vi "AnalogDAQ.vi"(0 "VISA resource name":refnum<visa-resource-name>="COM1", 1 "baud rate":u32=9600, 2 "data bits":u16=8 min=5 max=8 step=1, 3 "parity":u16(ring) items=["None", "Odd", "Even", "Mark", "Space"], 4 "stop bits":u16(ring)=10 items=["1.0"=10, "1.5"=15, "2.0"=20], 7 "flow control":u16(ring) items=["None"=0, "XON/XOFF"=1, "RTS/CTS"=2, "DTR/DSR"=4]) -> ()   [LabVIEW 2013]
doc: "The Basic Serial Read and Write example performs a Serial Port Read, a Serial Port Write, or a combination of these actions. The user selects the actions (read or write) on the front panel. If both are selected, the VI will write the data first, read data, and then close the VISA session that is opened to the port. This VI will wait until the specified number of bytes is received at the port. Only the number of bytes specified will be read.\n\nINSTRUCTIONS:\n1) Select the serial resource and configuration parameters (baud rate, data bits, parity, stop bits, flow control).\n2) Select the operations to be performed. \n3) Connect the serial port to your device. If no device is available, perform a loopback test by doing one of the following. Short pins 2 and 3 on a RS-232 cable or short pin 4 to pin 8 and pin 5 to pin 9 on a RS-485/422 cable. \n4) Run the VI to see the data read. (The \"read string\" will match the \"string to write\" if a loopback test was performed.)\n\nNote: The parameters set for the serial port must match the parameters of the connected instrument or device. In this example, the bytes to read parameter specifies the number of bytes that the serial port reads. If there were more bytes at the port than the number specified in bytes to read, those bytes would not be read. Also, if you specify to read more bytes than the number of bytes actually read, you might receive a timeout error message.\n\nOn the block diagram, the Configure Serial Port VI sets the configuration parameters. The front panel displays the controls used to configure the basic parameters, such as baud rate, data bits, and parity. Constants configure the other parameters the user probably does not need set. After the VISA Configure Serial Port VI opens the VISA session and configures the port, the VI passes the VISA resource name to other VIs that perform operations on that VISA resource. The VISA Write function sends a command to the serial device and the VISA Read function returns data based on the command. The VISA Close function then closes the reference to the serial device. It is important to close the reference; otherwise communication through with that port through protocols other than VISA might not be possible."
uses:
  <vilib>/Instr/_visa.llb/VISA Configure Serial Port (Instr).vi
panel:
  in  "Plot visible":bool[](array[boolean])=[TRUE, TRUE, TRUE, TRUE, TRUE, TRUE, TRUE]
  in  "stop":bool
  out "Analog Read":dbl[][](graph)
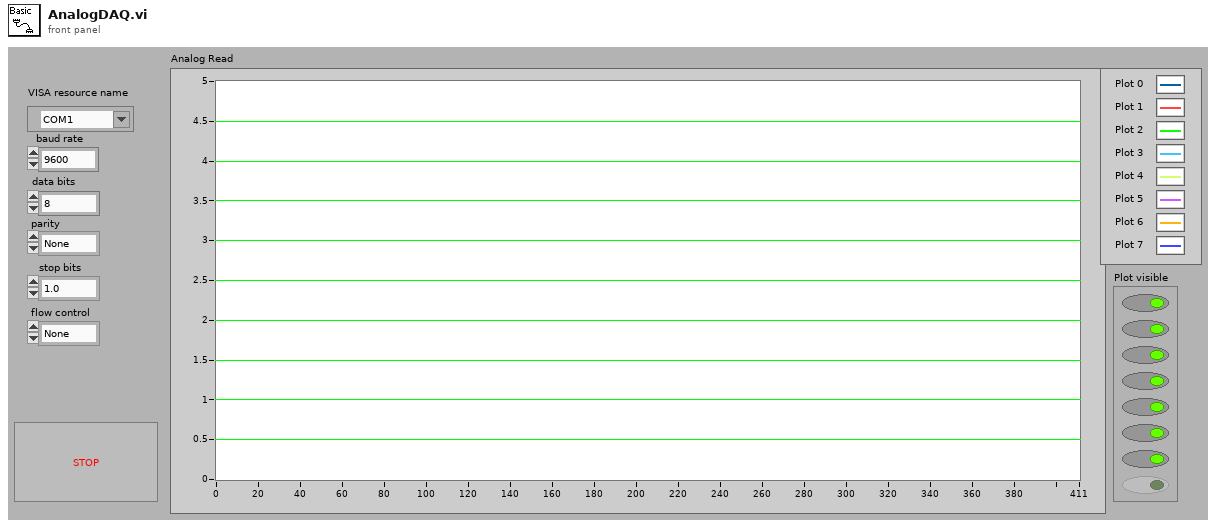
[diagram p1: front panel]
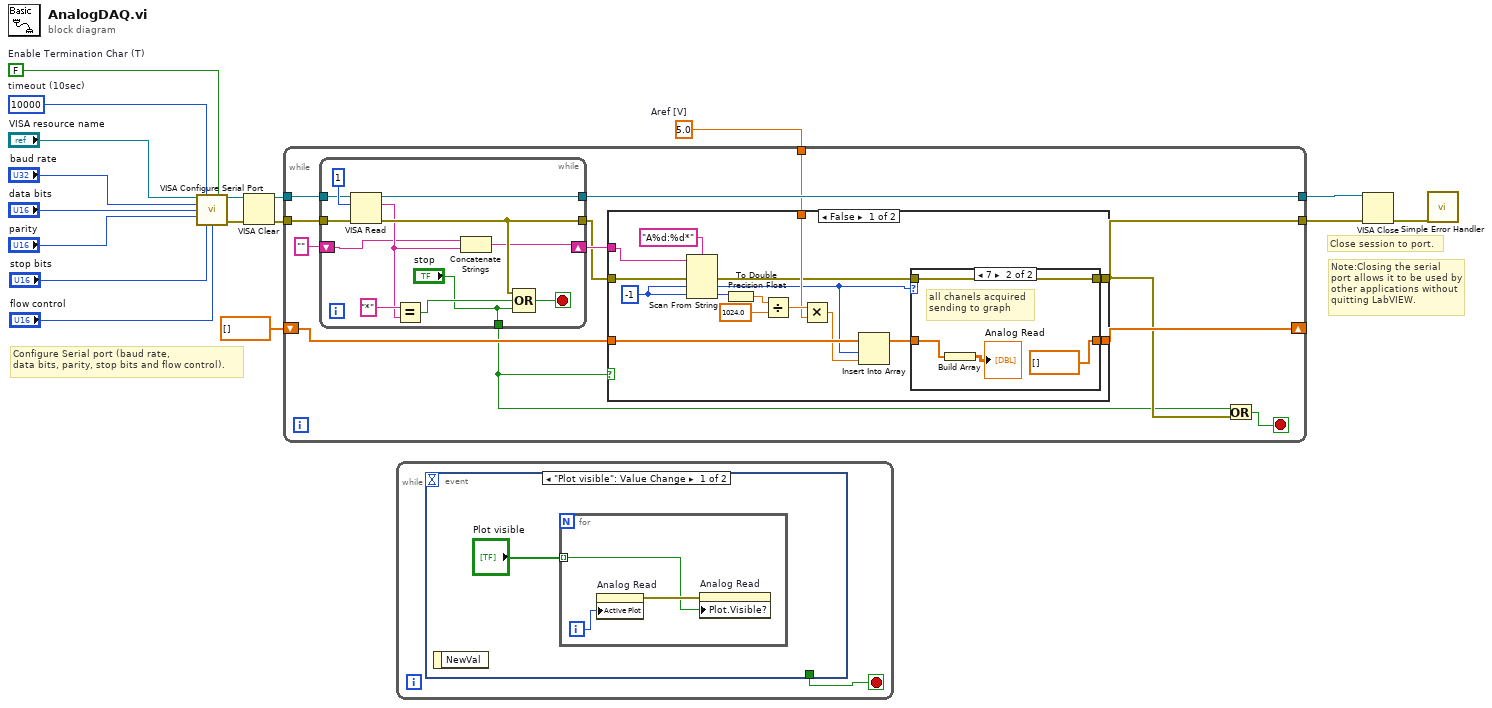
[diagram p0: block diagram]
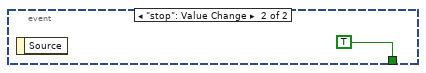
[diagram p2: hidden frame]
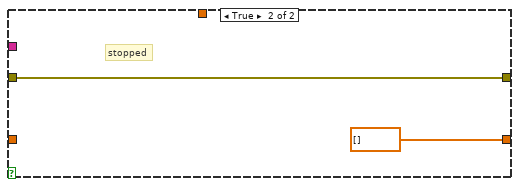
[diagram p4: hidden frame]
diagram:
  w5 = 5.0  # Aref [V]
  w12 = FALSE  # Enable Termination Char (T)
  w13 = u32 10000  # timeout (10sec)
  # "Note:Closing the serial port allows it to be used by other applications without\nquitting LabVIEW."
  # "Configure Serial port (baud rate,\ndata bits, parity, stop bits and flow control)."
  # "Close session to port."
  n1 = call-poly "VISA Configure Serial Port"("VISA resource name"="VISA resource name", "timeout (10sec)"=w13, "Enable Termination\nChar (T)"=w12, "baud rate (9600)"="baud rate", "data bits (8)"="data bits", "parity (0:none)"="parity", "stop bits (10: 1 bit)"="stop bits", "flow control (0:none)"="flow control") -> ("VISA resource name out"=w3:refnum<visa-resource-name>, "error out"=w4:errorcluster)  [unwired: 6 in]
  n2 = VISA Clear(VISA resource name=w3, error in (no error)=w4) -> (VISA resource name out=w2:refnum<visa-resource-name>, error out=w1:errorcluster)
  n3 = while {
    tunnel: [w19] -> w8
    tunnel: [w29] -> w7
    tunnel: w1 -> [w28]
    tunnel: w2 -> [w27]
    shift-right: [w20] -> _
    shift-left: dbl[] [] -> [w22]
    tunnel: w5 -> [w21]
    stop <- w25 stop-if-true
    n4 = while {
      tunnel: [w58] -> w23
      tunnel: [w65] -> w29
      tunnel: w28 -> [w63]
      tunnel: w27 -> [w62]
      shift-right: [w57] -> w24
      shift-left: "" -> [w55]
      tunnel: ["stop"] -> w18
      stop <- w59 stop-if-true
      n5 = VISA Read(VISA resource name=w62, byte count=u32 1 ("bytes to read 2"), error in (no error)=w63) -> (VISA resource name out=w65:refnum<visa-resource-name>, read buffer=w56:string, error out=w58:errorcluster)  [unwired: 1 out]
      n6 = Equal?(x="*", y=w56) -> (x = y?=w60:bool)
      n7 = Concatenate Strings(w55, w56) -> (w57:string)
      n8 = Compound Arithmetic op=OR(w58, w60, "stop") -> (w59:bool)
    }
    n9 = case shown="False" w18 {
      tunnel: w24 -> [w44 _]
      tunnel: w23 -> [w43 w52]
      tunnel: w22 -> [w41 _]
      tunnel: w21 -> [w36 _]
      tunnel: [w32 dbl[] []] -> w20
      tunnel: [w30 w52] -> w19
      frame False {
        w42 = -1 ("default value 1")
        n10 = Scan From String(format string="A%d:%d*", input string=w44, error in=w43, default 1=w42, default 2=w42) -> (error out=w31:errorcluster, output 1=w34:i32, output 2=w40:i32)  [unwired: 1 in, 2 out]
        n11 = To Double Precision Float(number=w40) -> (double precision float=w39:dbl)
        n12 = Divide(x=w39, y=1024.0) -> (x/y=w37:dbl)
        n13 = Multiply(x=w37, y=w36) -> (x*y=w35:dbl)
        n14 = Insert Into Array(array=w41, index=w34, new element=w35) -> (w33:dbl[])
        n15 = case shown="7" w34 {
          tunnel: w33 -> [w47 w48]
          tunnel: [w47 dbl[] []] -> w32
          tunnel: w31 -> [w46 w50]
          tunnel: [w46 w50] -> w30
          frame Default {
          }
          frame 7 {
            # "all chanels acquired\nsending to graph"
            n16 = Build Array(w48) -> (→"Analog Read":dbl[][])
          }
        }
      }
      frame True {
        # "stopped"
      }
    }
    n17 = Or(x=w18, y=w19) -> (x .or. y?=w25:bool)
  }
  n18 = while {
    stop <- w66 stop-if-true
    n19 = event shown="[0] \"Plot visible\": Value Change" {
      selector: _ -> [_ _]
      dyn-events: _ -> [_ _]
      timeout: _ -> [_ _]
      tunnel: [_ TRUE] -> w66
      event "Plot visible": Value Change {
        n20 = event-data() -> ()  [unwired: 1 in, 1 out]
        n21 = for {
          tunnel: "Plot visible" -> [w68] mode=indexing
          i -> [w70]
          n22 = property on="Analog Read" class="WFChart (strict)"("Active Plot"=w70) -> (error out=w69:errorcluster)  [unwired: 2 in, 1 out]
          n23 = property on="Analog Read" class="WFChart (strict)"(error in=w69, "Plot.Visible?"=w68) -> ()  [unwired: 1 in, 2 out]
        }
      }
      event "stop": Value Change {
        n24 = event-data() -> ()  [unwired: 1 in, 1 out]
      }
    }
  }
  n25 = VISA Close(VISA resource name=w7, error in (no error)=w8) -> (error out=w15:errorcluster)
  n26 = call <vilib>:"Simple Error Handler.vi"("error in (no error)"=w15) -> ()  [unwired: 4 in, 5 out]
